vi "Do.vi"(8 "error in (no error)":errorcluster, 9 "Events":refnum<class "Events.lvclass">, 10 "Message Loop Data in":T1, 11 "IInternalRequest in":refnum<class "HandlePublished JSON.lvclass">) -> (0 "error out":errorcluster, 2 "Message Loop Data out":T1, 3 "IInternalRequest out":refnum<class "HandlePublished JSON.lvclass">)   [LabVIEW 2020, in "wamplv.lvlib" / "HandlePublished JSON.lvclass"]
uses:
  HandlePublished JSON.lvclass
  HandlePublished JSON.lvclass/HandlePublished JSON.ctl
  WAMP Client/API/TypeDefs/Error or abort detail (JSON).ctl
  wamplv.lvlib
  WAMP Client/Private/TypeDef/PUBLISH result (JSON).ctl
  de862a02-472d-4984-ac9b-bcc25ffd4b17.vi
  <vilib>/ErrorRing/Error Ring.xnode
  <vilib>/Utility/error.llb/Error Cluster From Error Code.vi
  Publish/IPublish JSON/Publish JSON.lvclass
  Error/ErrorHandler JSON/ErrorHandler JSON.lvclass
  SerialisedMessages/JSONMessage/WampMessage JSON.lvclass
  C:/local/wamplv/Private/SerialisedMessages/JSONMessage/WampMessage JSON.lvclass
  C:/local/wamplv/Private/SerialisedMessages/IWampMessage/IWampMessage.lvclass
  WAMP Client/Private/TypeDef/Publish Requests Map.ctl
  WAMP Client/Private/TypeDef/Endpoint Data.ctl
  Call/ICallRequest/ICallRequest.lvclass
  WAMP Client/Private/TypeDef/CALL Request Map.ctl
  WAMP Client/Private/TypeDef/SUBSCRIBE Requests Map.ctl
  WAMP Client/Private/TypeDef/Subscriptions Map.ctl
  WAMP Client/Private/TypeDef/Unsubscribe Requests Map.ctl
  WAMP Client/Private/TypeDef/Unregister requests map.ctl
  WAMP Client/Private/TypeDef/Message Loop Data.ctl
  Events/EventsParent/Events.lvclass
  Subscribe/ISubscribe/ISubscribe.lvclass
  Publish/IPublish/IPublish.lvclass
  Message loop classes/Subscription details/SubscriptionDetailsParent/SubscriptionDetailsParent.lvclass
  Unsubscribe/IUnsubscribe/IUnsubscribe.lvclass
  Register/IRegister/IRegister.lvclass
  Unregister/IUnregister/IUnregister.lvclass
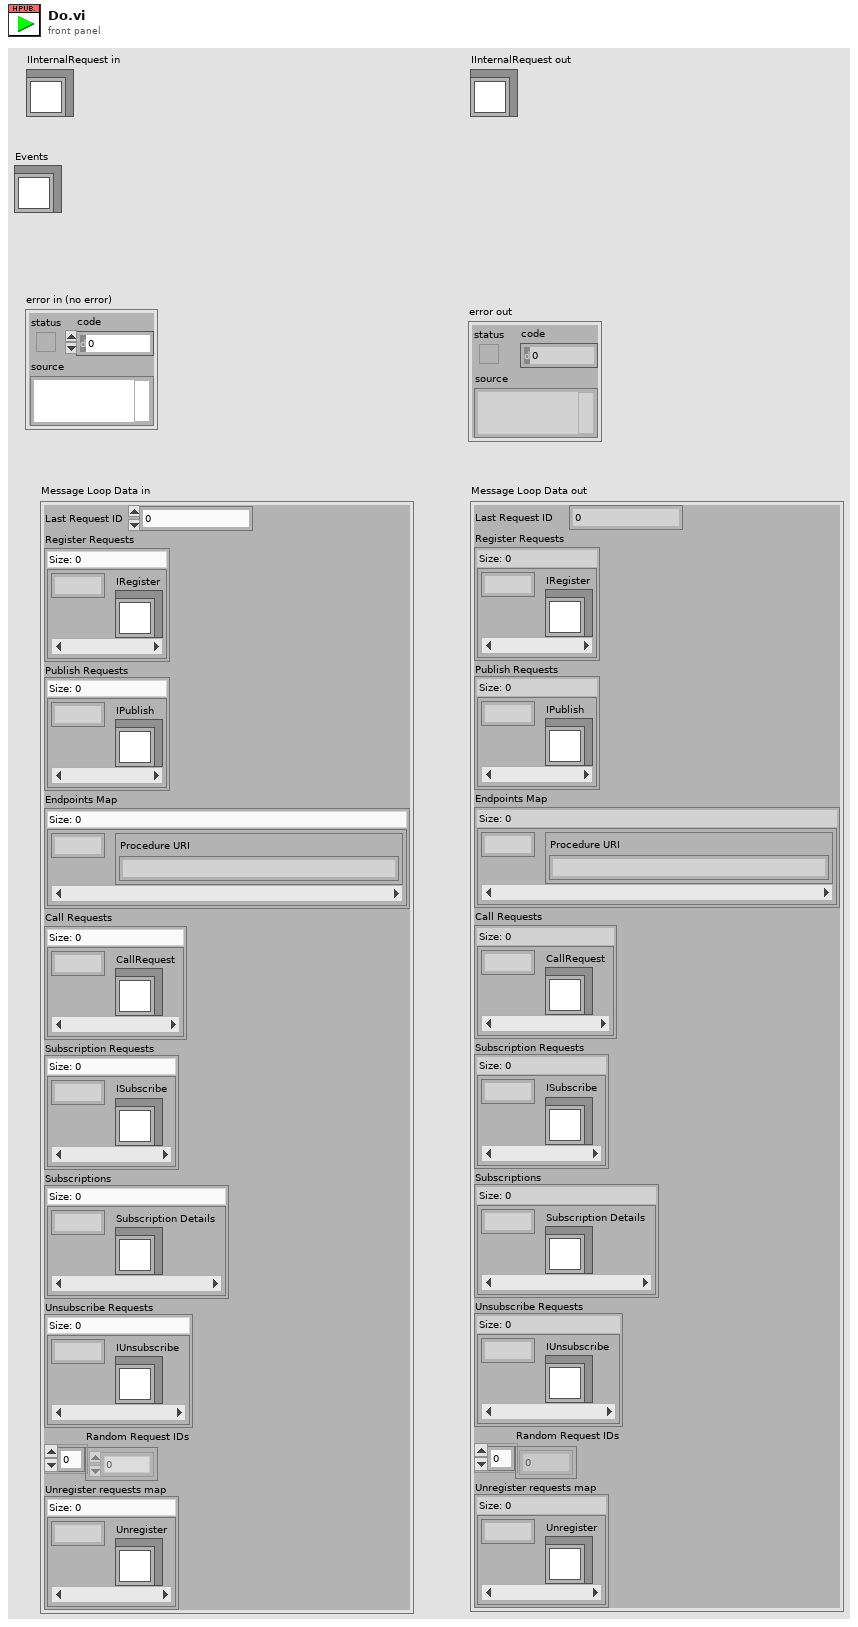
[diagram p1: front panel]
types:
  T1 = typedef "wamplv.lvlib/Message Loop Data.ctl" = cluster{"Last Request ID":u64, "Register Requests":map{u64, refnum<class "IRegister.lvclass">}, "Publish Requests":T2, "Endpoints Map":map{u64, T3}, "Call Requests":T4, "Subscription Requests":T5, "Subscriptions":T6, "Unsubscribe Requests":T7, "Random Request IDs":u64[], "Unregister requests map":T8}
  T2 = typedef "wamplv.lvlib/Publish Requests Map.ctl" = map{u64, refnum<class "IPublish.lvclass">}
  T3 = typedef "wamplv.lvlib/Endpoint Data.ctl" = cluster{"Procedure URI":string}
  T4 = typedef "wamplv.lvlib/CALL Request Map.ctl" = map{u64, refnum<class "ICallRequest.lvclass">}
  T5 = typedef "wamplv.lvlib/SUBSCRIBE Requests Map.ctl" = map{u64, refnum<class "ISubscribe.lvclass">}
  T6 = typedef "wamplv.lvlib/Subscriptions Map.ctl" = map{u64, refnum<class "SubscriptionDetailsParent.lvclass">}
  T7 = typedef "wamplv.lvlib/Unsubscribe Requests Map.ctl" = map{u64, refnum<class "IUnsubscribe.lvclass">}
  T8 = typedef "wamplv.lvlib/Unregister requests map.ctl" = map{u64, refnum<class "IUnregister.lvclass">}
  T9 = typedef "wamplv.lvlib/PUBLISH result (JSON).ctl" = cluster{"Publication ID":u64, "Success?":bool, "Error/Abort details (JSON)":T10}
  T10 = typedef "wamplv.lvlib/Error or abort detail (JSON).ctl" = cluster{"URI":string, "Arguments Payload":string, "ArgumentKw Payload":string, "Details":string, "Associated LabVIEW Error":errorcluster}
  T11 = typedef "wamplv.lvlib/WAMP Message Codes.ctl" = enum8{"HELLO", "WELCOME", "CHALLENGE", "AUTHENTICATE", "ABORT", "GOODBYE", "ERROR", "PUBLISH", "PUBLISHED", "SUBSCRIBE", "SUBSCRIBED", "UNSUBSCRIBE", "UNSUBSCRIBED", "EVENT", "CALL", "RESULT", "REGISTER", "REGISTERED", "UNREGISTER", "UNREGISTERED", "INVOCATION", "YIELD"}
  T12 = typedef "wamplv.lvlib/Error (JSON).ctl" = cluster{"Request ID":u64, "Message type that caused error":T11, "Error/Abort details (JSON)":T10}
  T13 = typedef "wamplv.lvlib/PUBLISH Request Data (JSON).ctl" = cluster{"Topic URI":string, "Arguments":string, "ArgumentsKw":string, "Request Acknowledgement":bool, "Options":string, "Publish result notifier":refnum<notifier>}
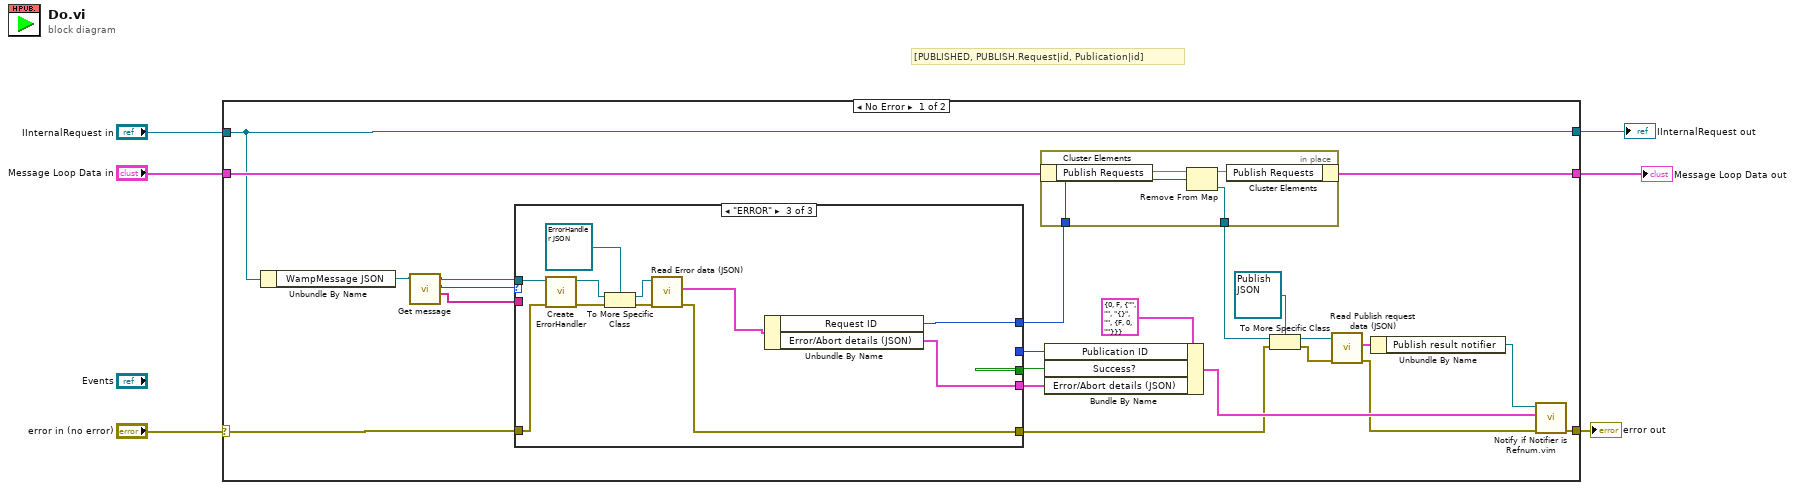
[diagram p0: block diagram]
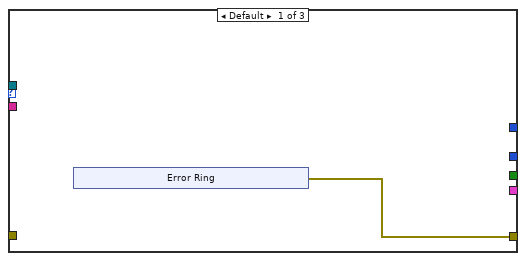
[diagram p2: hidden frame]
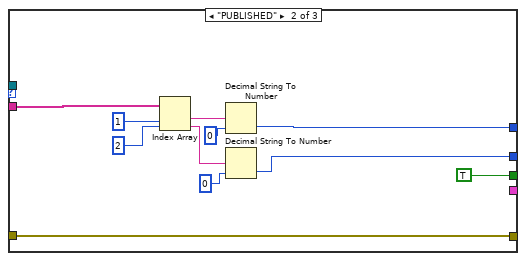
[diagram p3: hidden frame]
diagram:
  # "[PUBLISHED, PUBLISH.Request|id, Publication|id]"
  n1 = case shown="No Error" "error in (no error)" {
    selector: "error in (no error)" -> [w11 w61]
    tunnel: "Message Loop Data in" -> [w25 w62]
    tunnel: [w24 w62] -> w5
    tunnel: [w23 w61] -> w4
    tunnel: "IInternalRequest in" -> [w12 w63]
    tunnel: [w12 w63] -> w2
    frame No Error {
      n2 = Unbundle By Name(w12) -> ("WampMessage JSON"=w10:refnum<class "WampMessage JSON.lvclass">)
      n3 = call "Get message.vi"("JSONMessage in"=w10) -> ("<JSON>Elements"=w7:string[], "Message Type"=w8:T11, "JSONMessage out"=w9:refnum<class "WampMessage JSON.lvclass">)  [unwired: 8 in]
      n4 = case shown="\"ERROR\"" w8 {
        tunnel: w7 -> [_ w42 _]
        tunnel: [_ w44 w50] -> w27
        tunnel: w11 -> [_ w48 w59]
        tunnel: [w34 w48 w53] -> w19
        tunnel: [_ TRUE ("Success?") _] -> w29
        tunnel: w9 -> [_ _ w60]
        tunnel: [_ w41 _] -> w22
        tunnel: [_ _ w51] -> w18
        frame Default {
          n5 = xnode "Error Ring"() -> ("error out"=w34:errorcluster)
        }
        frame "PUBLISHED" {
          # "PUBLISHED"
          n6 = Index Array(array=w42, index #1=1 ("index"), index #2=2 ("index")) -> (element #1=w46:string, element #2=w39:string)
          n7 = Decimal String To Number(string=w46, default (0L)=u64 0) -> (number=w44:u64)  [unwired: 1 in, 1 out]
          n8 = Decimal String To Number(string=w39, default (0L)=u64 0) -> (number=w41:u64)  [unwired: 1 in, 1 out]
        }
        frame "ERROR" {
          # "ERROR"
          n9 = call "Create ErrorHandler.vi"("error in (no error)"=w59, "IWampMessage"=w60) -> ("error out"=w58:errorcluster, "IErrorHandler out"=w55:refnum<class "IErrorHandler.lvclass">)  [unwired: 8 in]
          n10 = To More Specific Class(target class=refnum<class "ErrorHandler JSON.lvclass"> refnum ("wamplv.lvlib:ErrorHandler JSON.lvclass"), reference=w55, error in=w58) -> (specific class reference=w54:refnum<class "ErrorHandler JSON.lvclass">, error out=w57:errorcluster)
          n11 = call "Read Error data (JSON).vi"("error in (no error)"=w57, "ErrorHandler JSON in"=w54) -> ("error out"=w53:errorcluster, "Error data (JSON)"=w52:T12)  [unwired: 7 in, 1 out]
          n12 = Unbundle By Name(w52) -> ("Request ID"=w50:u64, "Error/Abort details (JSON)"=w51:T10)
        }
      }
      n13 = in-place "In Place Element Structure" {
        in-place-border: w27 -> [w33]
        in-place-border: [w30] -> w20
        n14 = in-place-cluster #1(w25) -> ("Publish Requests"=w32:T2)
        n15 = Remove From Map(10:w33, 11:w32) -> (1:w30:refnum<class "IPublish.lvclass">, 3:w31:T2)  [unwired: 1 out]
        n16 = in-place-cluster #1("Publish Requests"=w31) -> (w24:T1)
      }
      n17 = Bundle By Name(cluster=T9 {"Publication ID"=0, "Success?"=FALSE, "Error/Abort details (JSON)"={"URI"="", "Arguments Payload"="", "ArgumentKw Payload"="{}", "Details"="", "Associated LabVIEW Error"={"status"=FALSE, "code"=0, "source"=""}}} ("Cluster"), "Publication ID"=w22, "Success?"=w29, "Error/Abort details (JSON)"=w18) -> (w26:T9)
      n18 = To More Specific Class(target class=refnum<class "Publish JSON.lvclass"> refnum ("wamplv.lvlib:Publish JSON.lvclass"), reference=w20, error in=w19) -> (specific class reference=w17:refnum<class "Publish JSON.lvclass">, error out=w14:errorcluster)
      n19 = call "Read Publish request data (JSON).vi"("error in (no error)"=w14, "Publish JSON in"=w17) -> ("error out"=w13:errorcluster, "Publish request data (JSON)"=w16:T13)  [unwired: 7 in, 1 out]
      n20 = Unbundle By Name(w16) -> ("Publish result notifier"=w15:refnum<notifier>)
      n21 = call "Notify if Notifier is Refnum.vim"("error in (no error)"=w13, "RESULT Payload"=w26, "Notifier in"=w15) -> ("error out"=w23:errorcluster)  [unwired: 8 in]
    }
    frame Error {
    }
  }
  "error out" <- w4
  "IInternalRequest out" <- w2
  "Message Loop Data out" <- w5
